vi "DAQ_Dig Freq Meas Configure and Measure.vi"(0 "DAQmx Task In":refnum<k21>, 5 "Range Settings":T1={"Max Frequency (Hz)"=20000000.0, "Min Frequency (Hz)"=1.0} {"Min Frequency (Hz)" format="%.6p"; "Max Frequency (Hz)" format="%.6p"}, 7 "Input Frequency Divisor":u32=4 min=4 step=1, 11 "error in":errorcluster) -> (4 "DAQmx Task Out":refnum<k21>, 6 "Detected Frequency (Hz)":dbl format="%.6p", 15 "error out":errorcluster)   [LabVIEW 2021, in "DAQ_Digital Frequency Measurement.lvlib"]
doc: "Configure, initiate and fetch digital frequency measurement from the channels configured."
uses:
  DAQ_Digital Frequency Measurement.lvlib
  Typedefs/Range Settings.ctl
  <vilib>/DAQmx/read.llb/DAQmx Read (Counter DBL 1Chan 1Samp).vi
  <vilib>/DAQmx/miscellaneous.llb/DAQmx Fill In Error Info.vi
  <resource>/objmgr/daqmx.rc
panel:
  # "Outputs"
  # "Inputs"
  # "Measurement Settings"
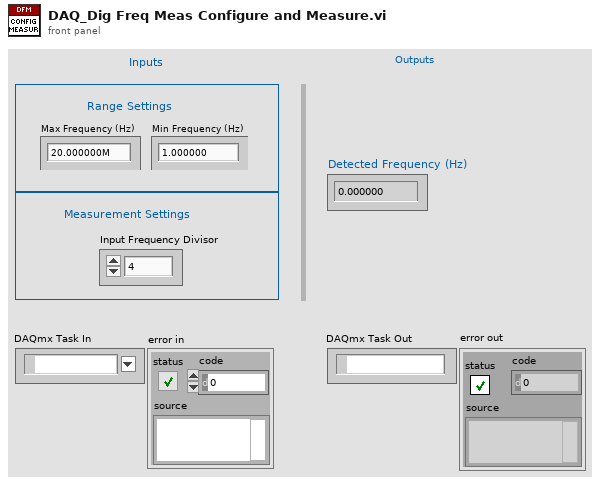
[diagram p1: front panel]
types:
  T1 = typedef "DAQ_Digital Frequency Measurement.lvlib/Range Settings.ctl" = cluster{"Max Frequency (Hz)":dbl, "Min Frequency (Hz)":dbl}
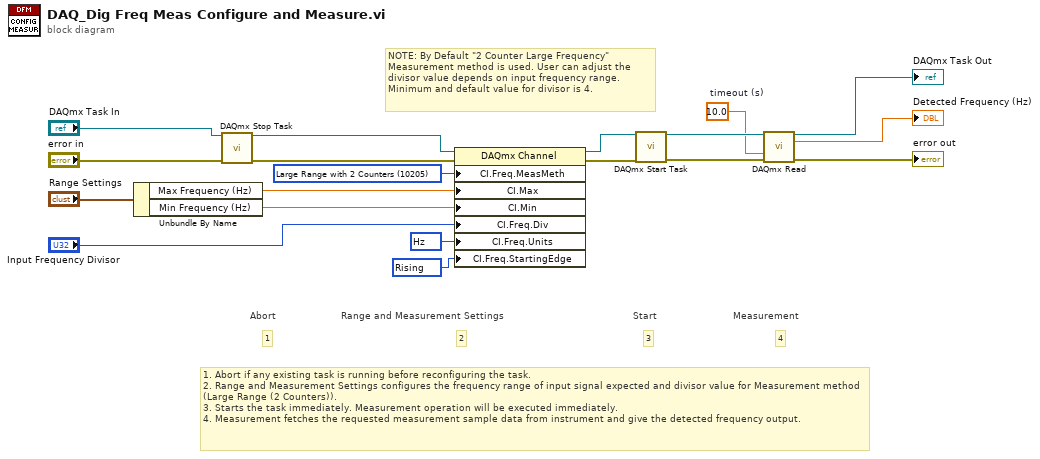
[diagram p0: block diagram]
diagram:
  w1 = 10280 items=["Rising"=10280, "Falling"=10171] ("CI.Freq.StartingEdge")
  w2 = 10373 items=["Hz"=10373, "Ticks"=10304, "From Custom Scale"=10065] ("CI.Freq.Units")
  w3 = 10205 items=["Low Frequency with 1 Counter"=10105, "High Frequency with 2 Counters"=10157, "Large Range with 2 Counters"=10205, "Dynamic Averaging"=16065] ("CI.Freq.MeasMeth")
  w12 = 10.0  # timeout (s)
  # "NOTE: By Default \"2 Counter Large Frequency\" Measurement method is used. User can adjust the divisor value depends on input frequency range. Minimum and default value for divisor is 4."
  # "4"
  # "Measurement"
  # "3"
  # "Start"
  # "1"
  # "Abort"
  # "2"
  # "Range and Measurement Settings"
  # "1. Abort if any existing task is running before reconfiguring the task.\n2. Range and Measurement Settings configures the frequency range of input signal expected and divisor value for Measurement method (Large Range (2 Counters)).\n3. Starts the task immediately. Measurement operation will be executed immediately.\n4. Measurement fetches the requested measurement sample data from instrument and give the detected frequency output."
  n1 = Unbundle By Name("Range Settings") -> ("Max Frequency (Hz)"=w4:dbl, "Min Frequency (Hz)"=w8:dbl)
  n2 = call <vilib>:"DAQmx Stop Task.vi"("task/channels in"="DAQmx Task In", "error in"="error in") -> ("task out"=w10:refnum<k21>, "error out"=w13:errorcluster)  [unwired: 12 in]
  n3 = property class="DAQmx Channel"(reference=w10, error in=w13, "CI.Freq.MeasMeth"=w3, "CI.Max"=w4, "CI.Min"=w8, "CI.Freq.Div"="Input Frequency Divisor", "CI.Freq.Units"=w2, "CI.Freq.StartingEdge"=w1) -> (reference out=w9:refnum<k21>, error out=w11:errorcluster)
  n4 = call <vilib>:"DAQmx Start Task.vi"("task/channels in"=w9, "error in"=w11) -> ("task out"=w18:refnum<k21>, "error out"=w19:errorcluster)  [unwired: 12 in]
  n5 = call-poly <vilib>:"DAQmx Read.vi"("task/channels in"=w18, "timeout"=w12, "error in"=w19) -> ("task out"=→"DAQmx Task Out":refnum<k21>, "data"=→"Detected Frequency (Hz)":dbl, "error out"=→"error out":errorcluster)  [unwired: 10 in]
